vi "File Footer Writer.vi"(6 "Old Data":dbl[][](array[numeric]), 9 "TDMS File Cluster":T1, 10 "Sample Rate":i32, 11 "In Use Cluster":T2) -> ()   [LabVIEW 2014]
panel:
  # "File Footer Writer VI"
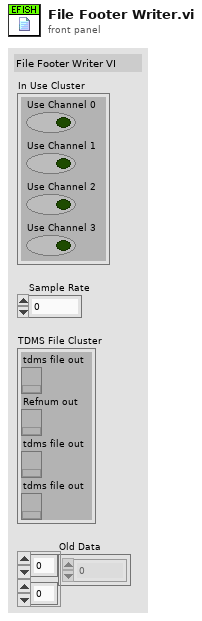
[diagram p1: front panel]
types:
  T1 = cluster{"tdms file out":refnum<k34>, "Refnum out":refnum<k34>, "tdms file out":refnum<k34>, "tdms file out":refnum<k34>}
  T2 = cluster{"Use Channel 0":bool, "Use Channel 1":bool, "Use Channel 2":bool, "Use Channel 3":bool}
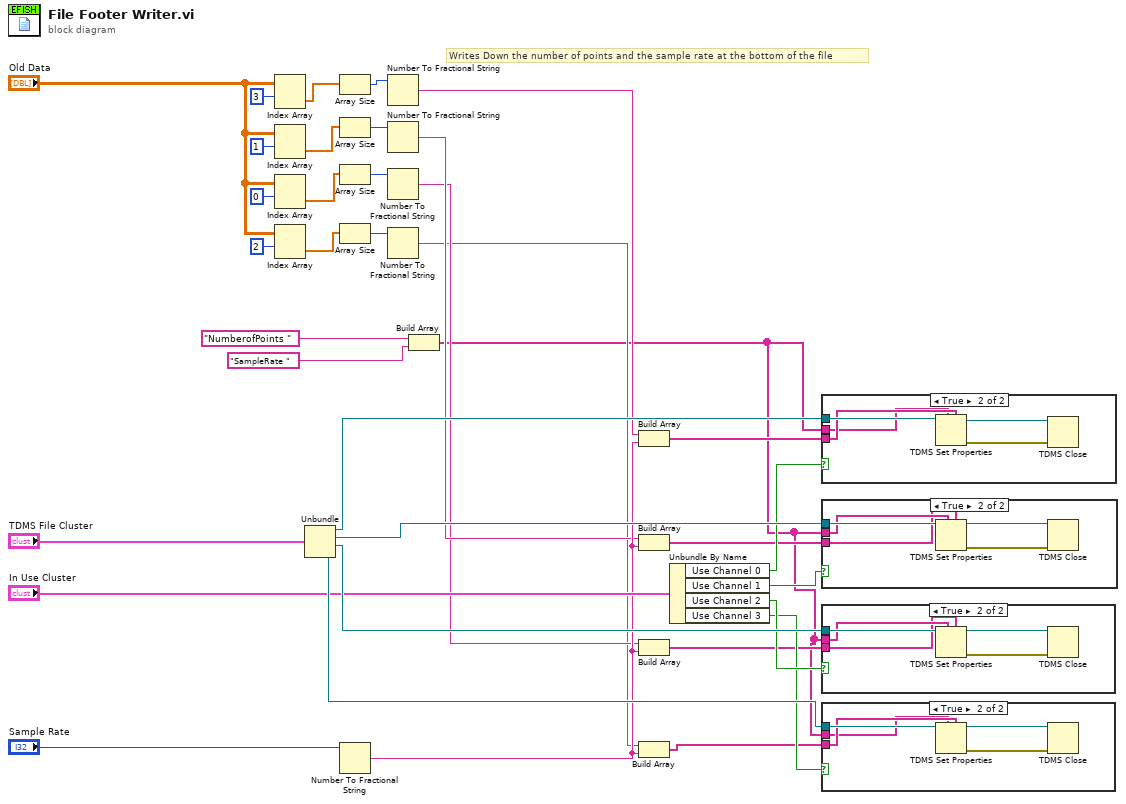
[diagram p0: block diagram]
diagram:
  # "Writes Down the number of points and the sample rate at the bottom of the file"
  n1 = Index Array(array="Old Data", index (row)=3) -> (element=w29:dbl[])  [unwired: 1 in]
  n2 = Index Array(array="Old Data", index (row)=1) -> (element=w31:dbl[])  [unwired: 1 in]
  n3 = Index Array(array="Old Data", index (row)=0) -> (element=w34:dbl[])  [unwired: 1 in]
  n4 = Index Array(array="Old Data", index (row)=2) -> (element=w36:dbl[])  [unwired: 1 in]
  n5 = Unbundle("TDMS File Cluster") -> ("tdms file out"=w25:refnum<k34>, "Refnum out"=w26:refnum<k34>, "tdms file out"=w27:refnum<k34>, "tdms file out"=w28:refnum<k34>)
  n6 = Array Size(array=w29) -> (size(s)=w30:i32)
  n7 = Array Size(array=w31) -> (size(s)=w32:i32)
  n8 = Array Size(array=w34) -> (size(s)=w33:i32)
  n9 = Array Size(array=w36) -> (size(s)=w35:i32)
  n10 = Number To Fractional String(number="Sample Rate") -> (F-format string=w10:string)  [unwired: 3 in]
  n11 = Number To Fractional String(number=w30) -> (F-format string=w9:string)  [unwired: 3 in]
  n12 = Number To Fractional String(number=w32) -> (F-format string=w8:string)  [unwired: 3 in]
  n13 = Number To Fractional String(number=w33) -> (F-format string=w7:string)  [unwired: 3 in]
  n14 = Number To Fractional String(number=w35) -> (F-format string=w6:string)  [unwired: 3 in]
  n15 = Build Array("NumberofPoints " ("string"), "SampleRate ") -> (w2:string[])
  n16 = Build Array(w9, w10) -> (w5:string[])
  n17 = Build Array(w8, w10) -> (w4:string[])
  n18 = Build Array(w7, w10) -> (w3:string[])
  n19 = Build Array(w6, w10) -> (w1:string[])
  n20 = Unbundle By Name("In Use Cluster") -> ("Use Channel 0"=w16:bool, "Use Channel 1"=w15:bool, "Use Channel 2"=w14:bool, "Use Channel 3"=w13:bool)
  n21 = case shown="True" w16 {
    tunnel: w25 -> [_ w41]
    tunnel: w2 -> [_ w37]
    tunnel: w5 -> [_ w38]
    frame False {
    }
    frame True {
      n22 = TDMS Set Properties(5:w38, 7:w37, 11:w41) -> (0:w39:errorcluster, 3:w40:refnum<k34>)  [unwired: 3 in, 2 out]
      n23 = TDMS Close(8:w39, 11:w40) -> ()  [unwired: 2 out]
    }
  }
  n24 = case shown="True" w15 {
    tunnel: w26 -> [_ w46]
    tunnel: w4 -> [_ w42]
    tunnel: w2 -> [_ w43]
    frame False {
    }
    frame True {
      n25 = TDMS Set Properties(5:w42, 7:w43, 11:w46) -> (0:w44:errorcluster, 3:w45:refnum<k34>)  [unwired: 3 in, 2 out]
      n26 = TDMS Close(8:w44, 11:w45) -> ()  [unwired: 2 out]
    }
  }
  n27 = case shown="True" w14 {
    tunnel: w27 -> [_ w51]
    tunnel: w3 -> [_ w47]
    tunnel: w2 -> [_ w48]
    frame False {
    }
    frame True {
      n28 = TDMS Set Properties(5:w47, 7:w48, 11:w51) -> (0:w49:errorcluster, 3:w50:refnum<k34>)  [unwired: 3 in, 2 out]
      n29 = TDMS Close(8:w49, 11:w50) -> ()  [unwired: 2 out]
    }
  }
  n30 = case shown="True" w13 {
    tunnel: w28 -> [_ w56]
    tunnel: w2 -> [_ w52]
    tunnel: w1 -> [_ w53]
    frame False {
    }
    frame True {
      n31 = TDMS Set Properties(5:w53, 7:w52, 11:w56) -> (0:w54:errorcluster, 3:w55:refnum<k34>)  [unwired: 3 in, 2 out]
      n32 = TDMS Close(8:w54, 11:w55) -> ()  [unwired: 2 out]
    }
  }
